vi "FSM.vi"() -> ()   [LabVIEW 2016]
panel:
  in  "Input array":dbl[](array[numeric])
  in  "Learning rate":dbl
  in  "Offset 2":dbl
  in  "Offset 1":dbl
  out "Random values generated":bool
  out "Training end":bool
  in  "Target 8":dbl
  in  "Target 7":dbl
  in  "Target 6":dbl
  in  "Target 5":dbl
  in  "Target 4":dbl
  in  "Target 3":dbl
  in  "Target 2":dbl
  in  "Target 1":dbl
  in  "Stop":bool
  in  "Training":bool
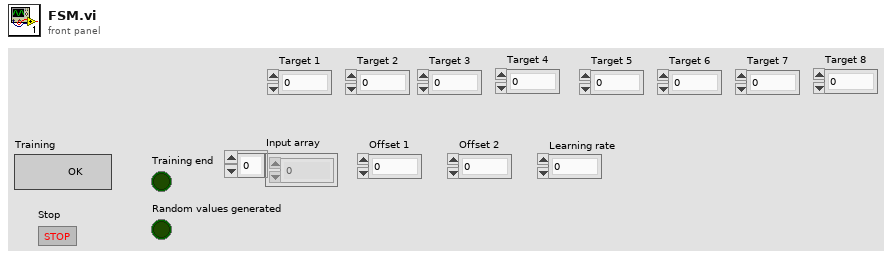
[diagram p1: front panel]
types:
  T1 = enum16{"Idle", "Generate weights", "Training mode", "Inference mode"}
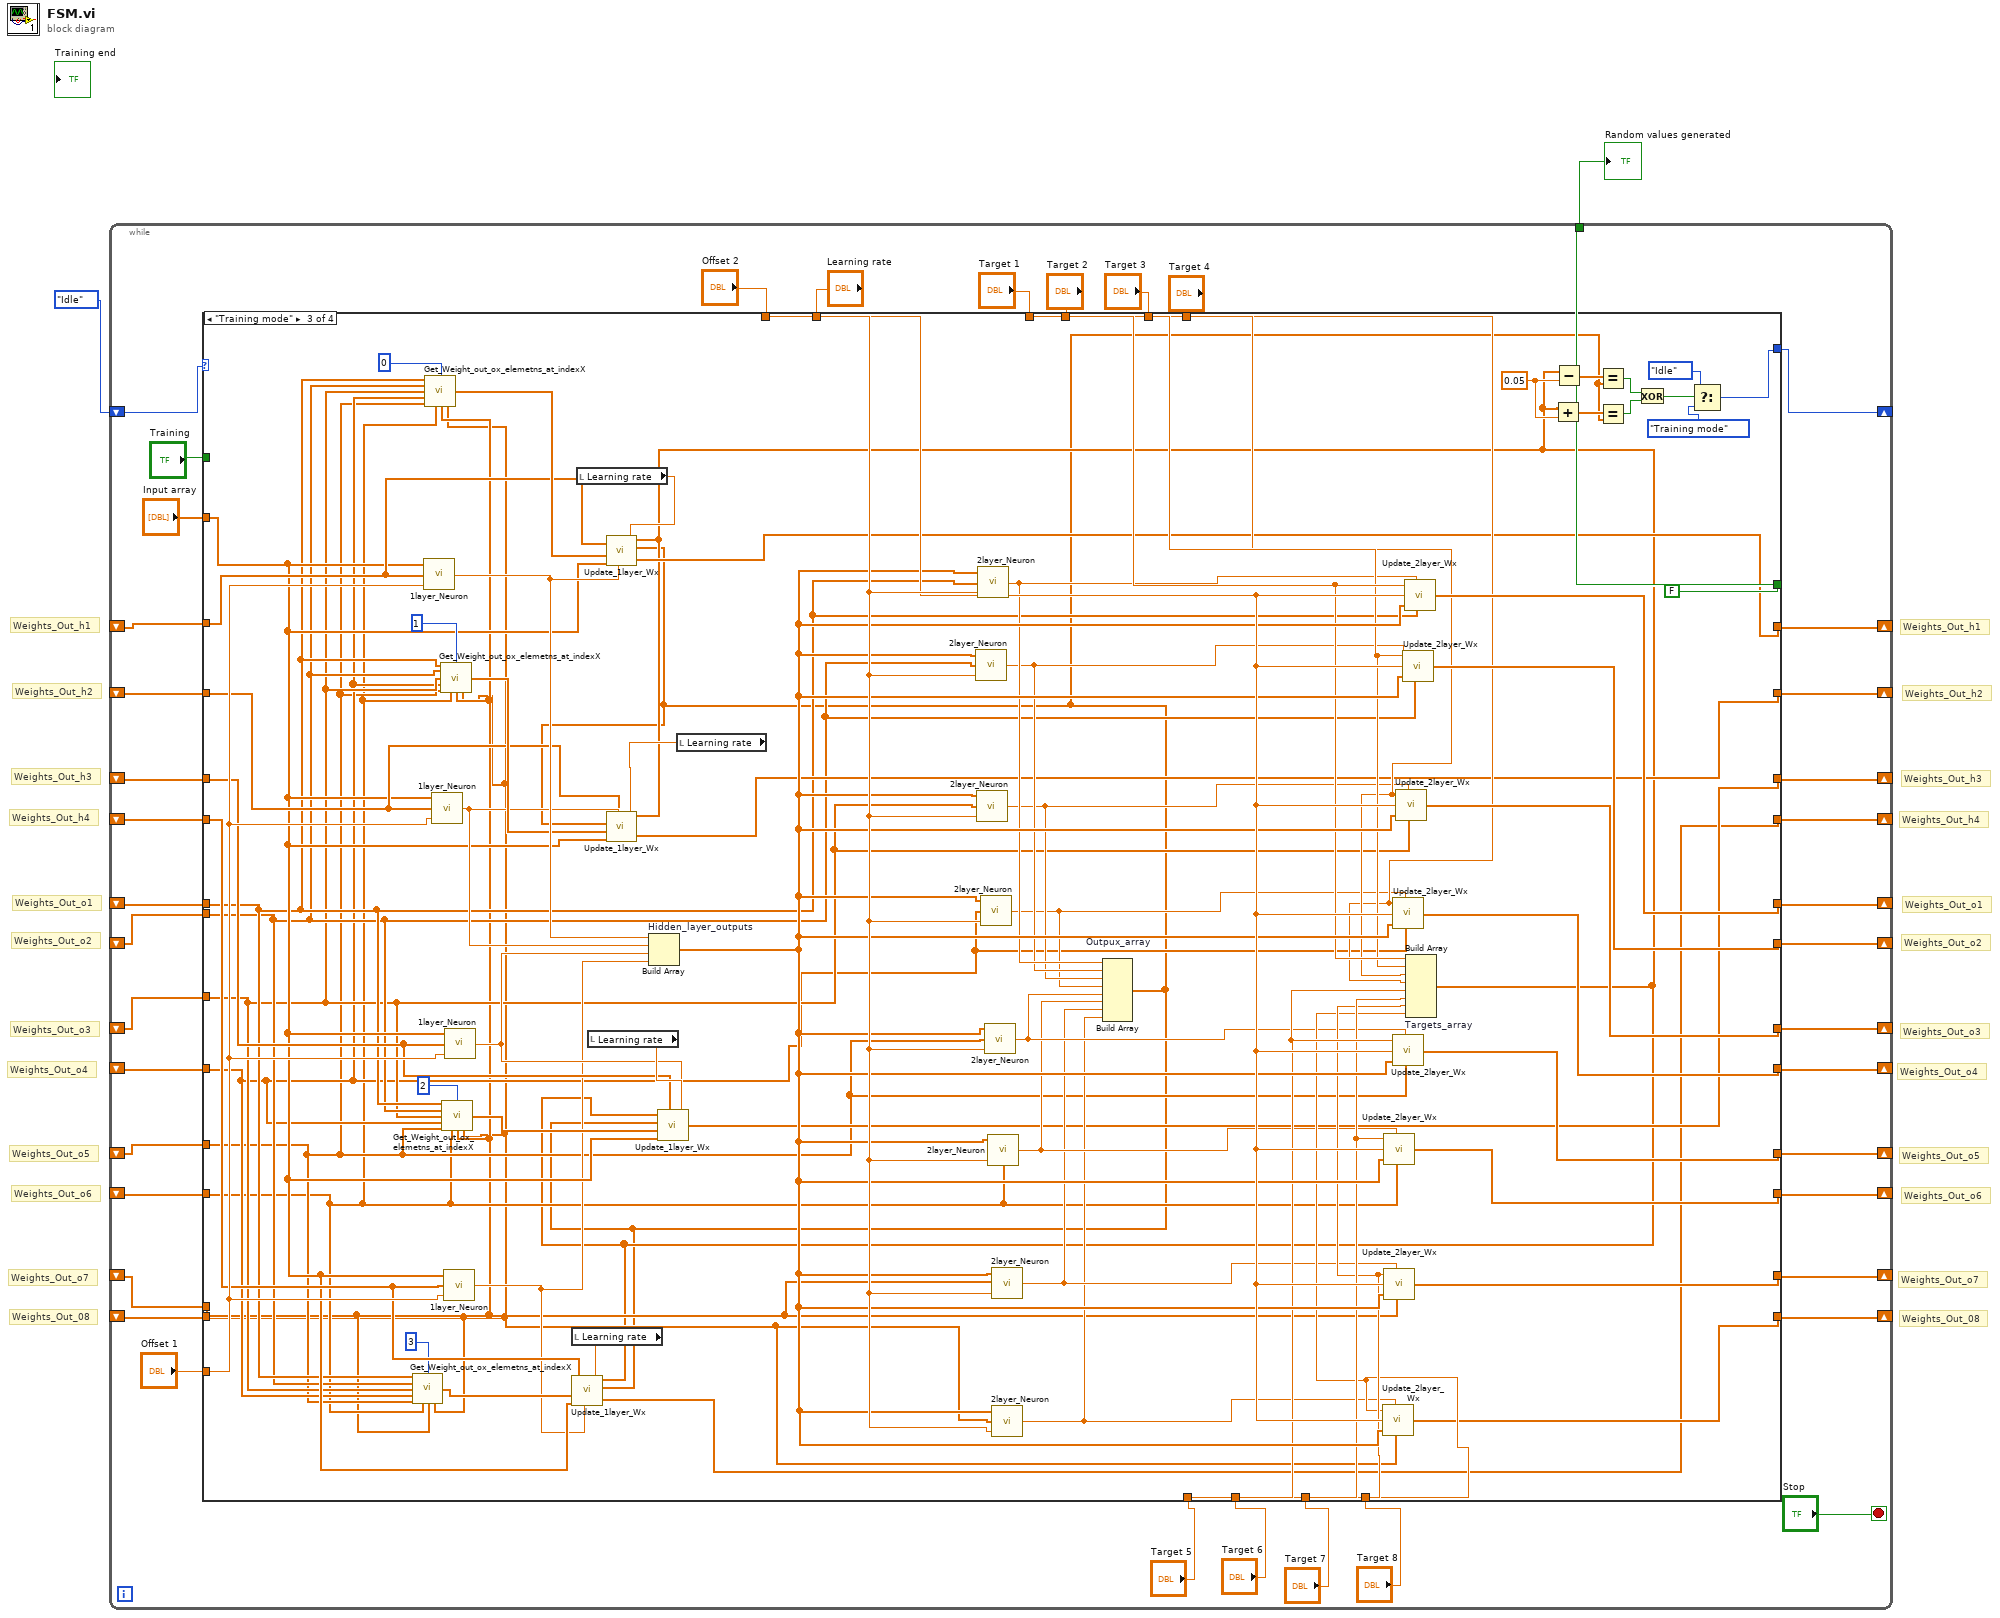
[diagram p0: block diagram]
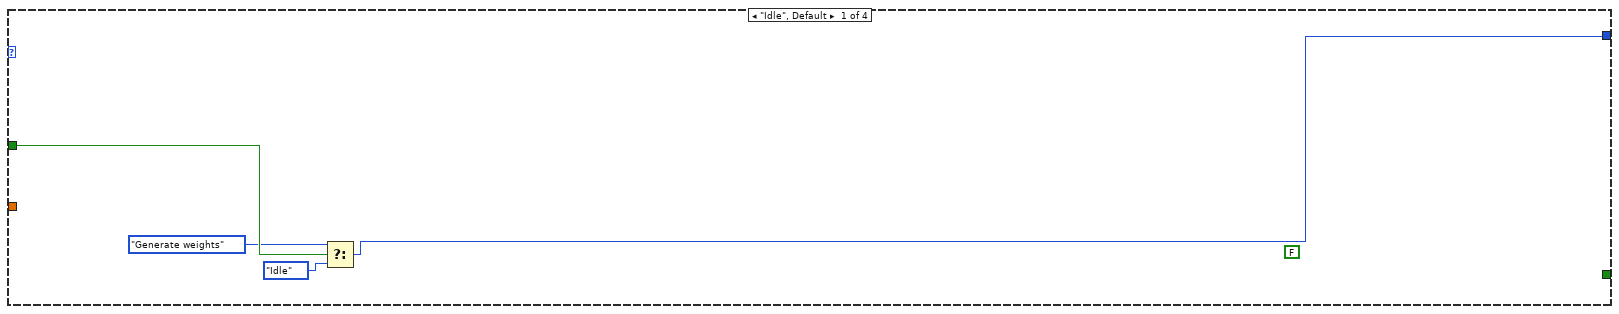
[diagram p2: hidden frame]
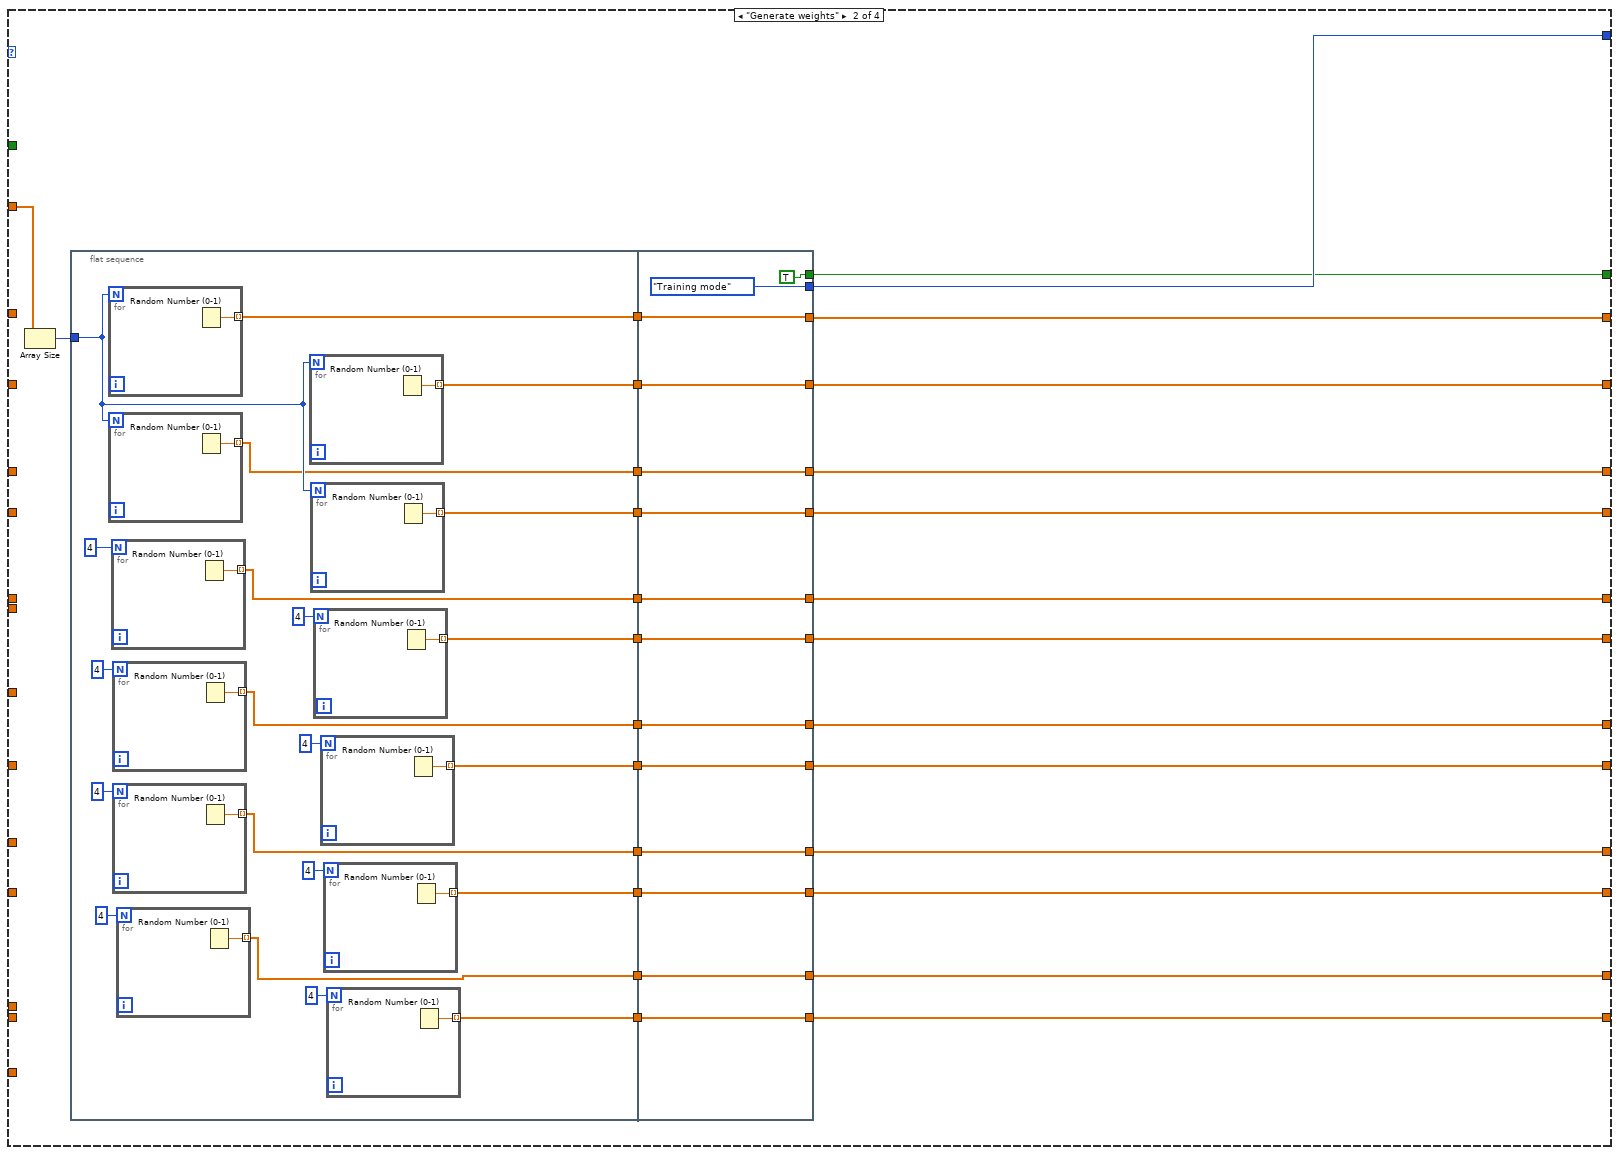
[diagram p3: hidden frame]
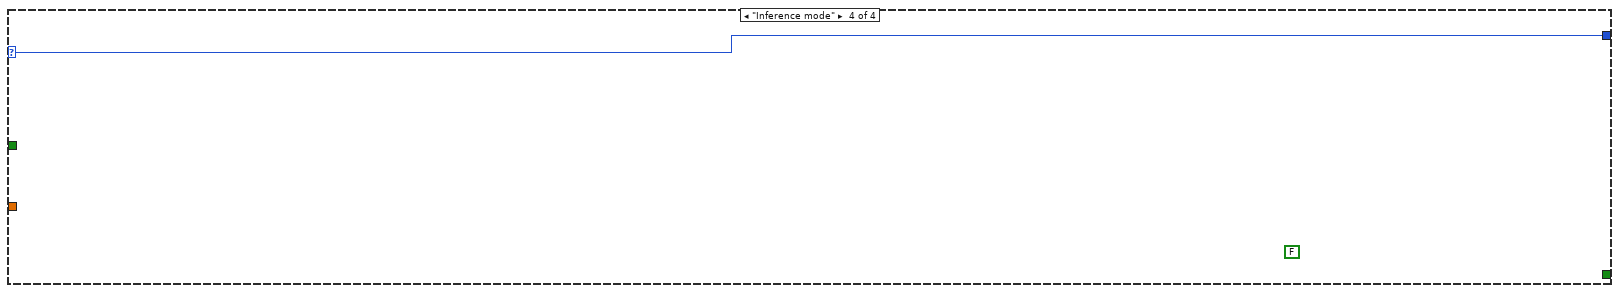
[diagram p4: hidden frame]
diagram:
  # "Weights_Out_08"
  # "Weights_Out_o7"
  # "Weights_Out_o5"
  # "Weights_Out_o6"
  # "Weights_Out_o4"
  # "Weights_Out_o3"
  # "Weights_Out_o2"
  # "Weights_Out_o1"
  # "Weights_Out_h4"
  # "Weights_Out_h3"
  # "Weights_Out_h2"
  # "Weights_Out_h1"
  # "Weights_Out_08"
  # "Weights_Out_o7"
  # "Weights_Out_o5"
  # "Weights_Out_o6"
  # "Weights_Out_o4"
  # "Weights_Out_o3"
  # "Weights_Out_o2"
  # "Weights_Out_o1"
  # "Weights_Out_h4"
  # "Weights_Out_h3"
  # "Weights_Out_h2"
  # "Weights_Out_h1"
  n1 = while {
    shift-right: [w3] -> _
    shift-left: T1."Idle" -> [w43]
    tunnel: [w41] -> w1
    shift-right: [w37] -> _
    shift-left: _ -> [w25]
    shift-right: [w36] -> _
    shift-left: _ -> [w24]
    shift-right: [w35] -> _
    shift-left: _ -> [w23]
    shift-right: [w34] -> _
    shift-left: _ -> [w22]
    shift-right: [w33] -> _
    shift-left: _ -> [w21]
    shift-right: [w32] -> _
    shift-left: _ -> [w16]
    shift-right: [w31] -> _
    shift-left: _ -> [w20]
    shift-right: [w30] -> _
    shift-left: _ -> [w19]
    shift-right: [w29] -> _
    shift-left: _ -> [w18]
    shift-right: [w28] -> _
    shift-left: _ -> [w17]
    shift-right: [w27] -> _
    shift-left: _ -> [w15]
    shift-right: [w26] -> _
    shift-left: _ -> [w14]
    stop <- "Stop" stop-if-true
    n2 = case shown="\"Training mode\"" w43 {
      selector: w43 -> [_ _ w124 w197]
      tunnel: "Training" -> [w47 _ _ _]
      tunnel: [w46 w75 w123 w197] -> w3
      tunnel: [_ w74 FALSE _] -> w41
      tunnel: "Offset 1" -> [_ _ w195 _]
      tunnel: "Offset 2" -> [_ _ w194 _]
      tunnel: "Input array" -> [_ w73 w146 _]
      tunnel: [_ w70 w162 _] -> w37
      tunnel: [_ w63 w156 _] -> w36
      tunnel: [_ w57 w150 _] -> w35
      tunnel: [_ w56 w135 _] -> w34
      tunnel: [_ w55 w191 _] -> w33
      tunnel: [_ w54 w190 _] -> w32
      tunnel: [_ w53 w189 _] -> w31
      tunnel: [_ w52 w188 _] -> w30
      tunnel: [_ w51 w187 _] -> w29
      tunnel: [_ w50 w186 _] -> w28
      tunnel: [_ w49 w185 _] -> w27
      tunnel: [_ w48 w168 _] -> w26
      tunnel: w25 -> [_ _ w163 _]
      tunnel: w24 -> [_ _ w158 _]
      tunnel: w23 -> [_ _ w153 _]
      tunnel: w22 -> [_ _ w148 _]
      tunnel: w21 -> [_ _ w143 _]
      tunnel: w16 -> [_ _ w142 _]
      tunnel: w20 -> [_ _ w141 _]
      tunnel: w19 -> [_ _ w140 _]
      tunnel: w18 -> [_ _ w139 _]
      tunnel: w17 -> [_ _ w138 _]
      tunnel: w15 -> [_ _ w137 _]
      tunnel: w14 -> [_ _ w136 _]
      tunnel: "Target 1" -> [_ _ w184 _]
      tunnel: "Learning rate" -> [_ _ w193 _]
      tunnel: "Target 2" -> [_ _ w183 _]
      tunnel: "Target 3" -> [_ _ w182 _]
      tunnel: "Target 4" -> [_ _ w181 _]
      tunnel: "Target 5" -> [_ _ w180 _]
      tunnel: "Target 6" -> [_ _ w179 _]
      tunnel: "Target 7" -> [_ _ w178 _]
      tunnel: "Target 8" -> [_ _ w177 _]
      frame "Idle", Default {
        (unwired) FALSE
        n3 = Select(t=T1."Generate weights", s=w47, f=T1."Idle") -> (s? t:f=w46:T1)
      }
      frame "Generate weights" {
        n4 = Array Size(array=w73) -> (size(s)=w72:i32)
        n5 = flat-sequence {
          tunnel: w72 -> [w96]
          tunnel: [w95] -> w71
          tunnel: [w94] -> w69
          tunnel: [w93] -> w68
          tunnel: [w92] -> w67
          tunnel: [w91] -> w66
          tunnel: [w90] -> w65
          tunnel: [w89] -> w64
          tunnel: [w88] -> w62
          tunnel: [w87] -> w61
          tunnel: [w86] -> w60
          tunnel: [w85] -> w59
          tunnel: [w84] -> w58
          tunnel: [T1."Training mode"] -> w75
          tunnel: [TRUE] -> w74
          tunnel: w71 -> [w120]
          tunnel: [w120] -> w70
          tunnel: w69 -> [w119]
          tunnel: [w119] -> w57
          tunnel: w68 -> [w118]
          tunnel: [w118] -> w55
          tunnel: w67 -> [w117]
          tunnel: [w117] -> w53
          tunnel: w66 -> [w116]
          tunnel: [w116] -> w51
          tunnel: w65 -> [w115]
          tunnel: [w115] -> w49
          tunnel: w64 -> [w114]
          tunnel: [w114] -> w63
          tunnel: w62 -> [w113]
          tunnel: [w113] -> w56
          tunnel: w61 -> [w112]
          tunnel: [w112] -> w54
          tunnel: w60 -> [w111]
          tunnel: [w111] -> w52
          tunnel: [w110] -> w50
          tunnel: w59 -> [w110]
          tunnel: w58 -> [w109]
          tunnel: [w109] -> w48
          frame #0 {
            n6 = for {
              N: w96 -> [_]
              tunnel: [w108] -> w95 mode=indexing
              n7 = Random Number (0-1)() -> (number: 0 to 1=w108:dbl)
            }
            n8 = for {
              N: w96 -> [_]
              tunnel: [w107] -> w94 mode=indexing
              n9 = Random Number (0-1)() -> (number: 0 to 1=w107:dbl)
            }
            n10 = for {
              N: 4 -> [_]
              tunnel: [w106] -> w93 mode=indexing
              n11 = Random Number (0-1)() -> (number: 0 to 1=w106:dbl)
            }
            n12 = for {
              N: 4 -> [_]
              tunnel: [w102] -> w92 mode=indexing
              n13 = Random Number (0-1)() -> (number: 0 to 1=w102:dbl)
            }
            n14 = for {
              N: 4 -> [_]
              tunnel: [w104] -> w91 mode=indexing
              n15 = Random Number (0-1)() -> (number: 0 to 1=w104:dbl)
            }
            n16 = for {
              N: 4 -> [_]
              tunnel: [w105] -> w90 mode=indexing
              n17 = Random Number (0-1)() -> (number: 0 to 1=w105:dbl)
            }
            n18 = for {
              N: w96 -> [_]
              tunnel: [w103] -> w89 mode=indexing
              n19 = Random Number (0-1)() -> (number: 0 to 1=w103:dbl)
            }
            n20 = for {
              N: w96 -> [_]
              tunnel: [w101] -> w88 mode=indexing
              n21 = Random Number (0-1)() -> (number: 0 to 1=w101:dbl)
            }
            n22 = for {
              N: 4 -> [_]
              tunnel: [w100] -> w87 mode=indexing
              n23 = Random Number (0-1)() -> (number: 0 to 1=w100:dbl)
            }
            n24 = for {
              N: 4 -> [_]
              tunnel: [w99] -> w86 mode=indexing
              n25 = Random Number (0-1)() -> (number: 0 to 1=w99:dbl)
            }
            n26 = for {
              N: 4 -> [_]
              tunnel: [w98] -> w85 mode=indexing
              n27 = Random Number (0-1)() -> (number: 0 to 1=w98:dbl)
            }
            n28 = for {
              N: 4 -> [_]
              tunnel: [w97] -> w84 mode=indexing
              n29 = Random Number (0-1)() -> (number: 0 to 1=w97:dbl)
            }
          }
          frame #1 {
          }
        }
      }
      frame "Training mode" {
        w134 = 0.05 ("x")
        n30 = call "Get_Weight_out_ox_elemetns_at_indexX.vi"("Array_Weight_Out_o1"=w143, "Index"=3, "Array_Weight_Out_o2"=w142, "Array_Weight_Out_o3"=w141, "Array_Weight_Out_o4"=w140, "Array_Weight_Out_o5"=w139, "Array_Weight_Out_o6"=w138, "Array_Weight_Out_o7"=w137, "Array_Weight_Out_o8"=w136) -> ("Output_array"=w147:dbl[])  [unwired: 6 in]
        n31 = call "1layer_Neuron.vi"("Offset"=w195, "Weights"=w163, "Inputs"=w146) -> ("Output"=w165:dbl)
        n32 = call "Get_Weight_out_ox_elemetns_at_indexX.vi"("Array_Weight_Out_o1"=w143, "Index"=0, "Array_Weight_Out_o2"=w142, "Array_Weight_Out_o3"=w141, "Array_Weight_Out_o4"=w140, "Array_Weight_Out_o5"=w139, "Array_Weight_Out_o6"=w138, "Array_Weight_Out_o7"=w137, "Array_Weight_Out_o8"=w136) -> ("Output_array"=w166:dbl[])  [unwired: 6 in]
        n33 = call "1layer_Neuron.vi"("Offset"=w195, "Weights"=w158, "Inputs"=w146) -> ("Output"=w159:dbl)
        n34 = call "Get_Weight_out_ox_elemetns_at_indexX.vi"("Array_Weight_Out_o1"=w143, "Index"=1, "Array_Weight_Out_o2"=w142, "Array_Weight_Out_o3"=w141, "Array_Weight_Out_o4"=w140, "Array_Weight_Out_o5"=w139, "Array_Weight_Out_o6"=w138, "Array_Weight_Out_o7"=w137, "Array_Weight_Out_o8"=w136) -> ("Output_array"=w160:dbl[])  [unwired: 6 in]
        n35 = call "Get_Weight_out_ox_elemetns_at_indexX.vi"("Array_Weight_Out_o1"=w143, "Index"=2, "Array_Weight_Out_o2"=w142, "Array_Weight_Out_o3"=w141, "Array_Weight_Out_o4"=w140, "Array_Weight_Out_o5"=w139, "Array_Weight_Out_o6"=w138, "Array_Weight_Out_o7"=w137, "Array_Weight_Out_o8"=w136) -> ("Output_array"=w152:dbl[])  [unwired: 6 in]
        n36 = call "1layer_Neuron.vi"("Offset"=w195, "Weights"=w148, "Inputs"=w146) -> ("Output"=w145:dbl)
        n37 = call "1layer_Neuron.vi"("Offset"=w195, "Weights"=w153, "Inputs"=w146) -> ("Output"=w151:dbl)
        n38 = local read "Learning rate"() -> (w149:dbl)
        n39 = local read "Learning rate"() -> (w164:dbl)
        n40 = local read "Learning rate"() -> (w155:dbl)
        n41 = Build Array "Hidden_layer_outputs"(w165, w159, w151, w145) -> (w192:dbl[])
        n42 = local read "Learning rate"() -> (w161:dbl)
        n43 = call "2layer_Neuron.vi"("Offset"=w194, "Weights_2layer"=w142, "Array_Out_hx"=w192) -> ("Output"=w175:dbl)
        n44 = call "2layer_Neuron.vi"("Offset"=w194, "Weights_2layer"=w141, "Array_Out_hx"=w192) -> ("Output"=w174:dbl)
        n45 = call "2layer_Neuron.vi"("Offset"=w194, "Weights_2layer"=w143, "Array_Out_hx"=w192) -> ("Output"=w176:dbl)
        n46 = call "2layer_Neuron.vi"("Offset"=w194, "Weights_2layer"=w140, "Array_Out_hx"=w192) -> ("Output"=w173:dbl)
        n47 = call "2layer_Neuron.vi"("Offset"=w194, "Weights_2layer"=w139, "Array_Out_hx"=w192) -> ("Output"=w172:dbl)
        n48 = call "2layer_Neuron.vi"("Offset"=w194, "Weights_2layer"=w138, "Array_Out_hx"=w192) -> ("Output"=w171:dbl)
        n49 = call "2layer_Neuron.vi"("Offset"=w194, "Weights_2layer"=w137, "Array_Out_hx"=w192) -> ("Output"=w170:dbl)
        n50 = call "2layer_Neuron.vi"("Offset"=w194, "Weights_2layer"=w136, "Array_Out_hx"=w192) -> ("Output"=w169:dbl)
        n51 = Build Array "Outpux_array"(w176, w175, w174, w173, w172, w171, w170, w169) -> (w130:dbl[])
        n52 = call "Update_2layer_Wx.vi"("Target_OutX"=w177, "2layer_OutX 2"=w169, "Learning rate"=w193, "Array_Out_hx"=w192, "Weights_2layer"=w136) -> ("Weights_2layer_updated"=w168:dbl[])
        n53 = call "Update_2layer_Wx.vi"("Target_OutX"=w179, "2layer_OutX 2"=w171, "Learning rate"=w193, "Array_Out_hx"=w192, "Weights_2layer"=w138) -> ("Weights_2layer_updated"=w186:dbl[])
        n54 = call "Update_2layer_Wx.vi"("Target_OutX"=w178, "2layer_OutX 2"=w170, "Learning rate"=w193, "Array_Out_hx"=w192, "Weights_2layer"=w137) -> ("Weights_2layer_updated"=w185:dbl[])
        n55 = call "Update_2layer_Wx.vi"("Target_OutX"=w181, "2layer_OutX 2"=w173, "Learning rate"=w193, "Array_Out_hx"=w192, "Weights_2layer"=w140) -> ("Weights_2layer_updated"=w188:dbl[])
        n56 = call "Update_2layer_Wx.vi"("Target_OutX"=w180, "2layer_OutX 2"=w172, "Learning rate"=w193, "Array_Out_hx"=w192, "Weights_2layer"=w139) -> ("Weights_2layer_updated"=w187:dbl[])
        n57 = call "Update_2layer_Wx.vi"("Target_OutX"=w182, "2layer_OutX 2"=w174, "Learning rate"=w193, "Array_Out_hx"=w192, "Weights_2layer"=w141) -> ("Weights_2layer_updated"=w189:dbl[])
        n58 = call "Update_2layer_Wx.vi"("Target_OutX"=w183, "2layer_OutX 2"=w175, "Learning rate"=w193, "Array_Out_hx"=w192, "Weights_2layer"=w142) -> ("Weights_2layer_updated"=w190:dbl[])
        n59 = call "Update_2layer_Wx.vi"("Target_OutX"=w184, "2layer_OutX 2"=w176, "Learning rate"=w193, "Array_Out_hx"=w192, "Weights_2layer"=w143) -> ("Weights_2layer_updated"=w191:dbl[])
        n60 = Build Array "Targets_array"(w184, w183, w182, w181, w180, w179, w178, w177) -> (w133:dbl[])
        n61 = call "Update_1layer_Wx.vi"("Learning rate"=w149, "1layer_Out_hx"=w145, "Array_Weights_hx"=w148, "Array_Inputs"=w146, "Array_2layer_Weights_at_Index_hx"=w147, "Array_Out_ox"=w130, "Array_target_ox"=w133) -> ("Array_Weights_hx_updated"=w135:dbl[])
        n62 = call "Update_1layer_Wx.vi"("Learning rate"=w164, "1layer_Out_hx"=w165, "Array_Weights_hx"=w163, "Array_Inputs"=w146, "Array_2layer_Weights_at_Index_hx"=w166, "Array_Out_ox"=w130, "Array_target_ox"=w133) -> ("Array_Weights_hx_updated"=w162:dbl[])
        n63 = call "Update_1layer_Wx.vi"("Learning rate"=w161, "1layer_Out_hx"=w159, "Array_Weights_hx"=w158, "Array_Inputs"=w146, "Array_2layer_Weights_at_Index_hx"=w160, "Array_Out_ox"=w130, "Array_target_ox"=w133) -> ("Array_Weights_hx_updated"=w156:dbl[])
        n64 = call "Update_1layer_Wx.vi"("Learning rate"=w155, "1layer_Out_hx"=w151, "Array_Weights_hx"=w153, "Array_Inputs"=w146, "Array_2layer_Weights_at_Index_hx"=w152, "Array_Out_ox"=w130, "Array_target_ox"=w133) -> ("Array_Weights_hx_updated"=w150:dbl[])
        n65 = Add(x=w133, y=w134) -> (x+y=w131:dbl[])
        n66 = Subtract(x=w133, y=w134) -> (x-y=w132:dbl[])
        n67 = Equal?(x=w132, y=w130) -> (x = y?=w129:bool)
        n68 = Equal?(x=w131, y=w130) -> (x = y?=w128:bool)
        n69 = Exclusive Or(1:w128, 2:w129) -> (0:w127:bool)
        n70 = Select(t=T1."Idle", s=w127, f=T1."Training mode") -> (s? t:f=w123:T1)
      }
      frame "Inference mode" {
        (unwired) FALSE
      }
    }
  }
  "Random values generated" <- w1
